vi "conversion 2.vi"(11 "Voltage":dbl=0.1 min=0.1 max=3.2 step=0.1) -> (3 "Distance (cm)":dbl)   [LabVIEW 2014]
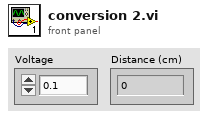
[diagram p1: front panel]
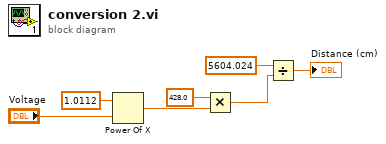
[diagram p0: block diagram]
diagram:
  n1 = Power Of X(1:"Voltage", 2:1.0112 ("x")) -> (0:w6:dbl)
  n2 = Multiply(x=428.0, y=w6) -> (x*y=w2:dbl)
  n3 = Divide(x=5604.024 ("y"), y=w2) -> (x/y=→"Distance (cm)":dbl)
